vi "Run.vi"(7 "Team Index":i32, 8 "Column":i32, 9 "Row":i32, 10 "View":i32[](array[numeric]) caption="View (Team Index, -1: empty)", 11 "Impenetrable In":refnum<class "Impenetrable.lvclass">) -> (0 "Replicated":refnum<class "Square.lvclass">, 1 "Direction":T1, 2 "Action":T2, 3 "Square Out":refnum<class "Square.lvclass">)   [LabVIEW 2015, in "Impenetrable.lvclass"]
uses:
  Impenetrable.lvclass
  Square/Square.lvclass
  Type Defs/Action Enum.ctl
  Type Defs/Direction Enum.ctl
  Impenetrable.lvclass/Impenetrable.ctl
  Assassin/Assassin.lvclass
  Type.ctl
  SubVIs/Read-Only Globals.vi
  Common/Find Enemy.vi
  SubVIs/Globals (private).vi
  Globals.vi
  Common/Common.lvlib
  Type Defs/SB Type Defs.lvlib
panel:
  # "NW\nN\nNE\nE\nSE\nS\nSW\nW"
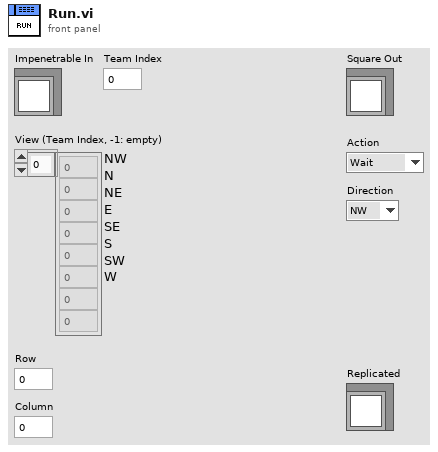
[diagram p1: front panel]
types:
  T1 = typedef "SB Type Defs.lvlib/Direction Enum.ctl" = enum16{"NW", "N", "NE", "E", "SE", "S", "SW", "W"}
  T2 = typedef "SB Type Defs.lvlib/Action Enum.ctl" = enum16{"Wait", "Move", "Attack", "Replicate"}
  T3 = typedef "Impenetrable.lvclass/Type.ctl" = enum16{"Assassin", "Starter", "Line Starter", "ELine", "WLine", "StartPatrol", "WPatrol", "EPatrol", "WWall", "EWall", "Rain"}
  T4 = typedef "Common.lvlib/Position.ctl" = cluster{"Column":i32, "Row":i32}
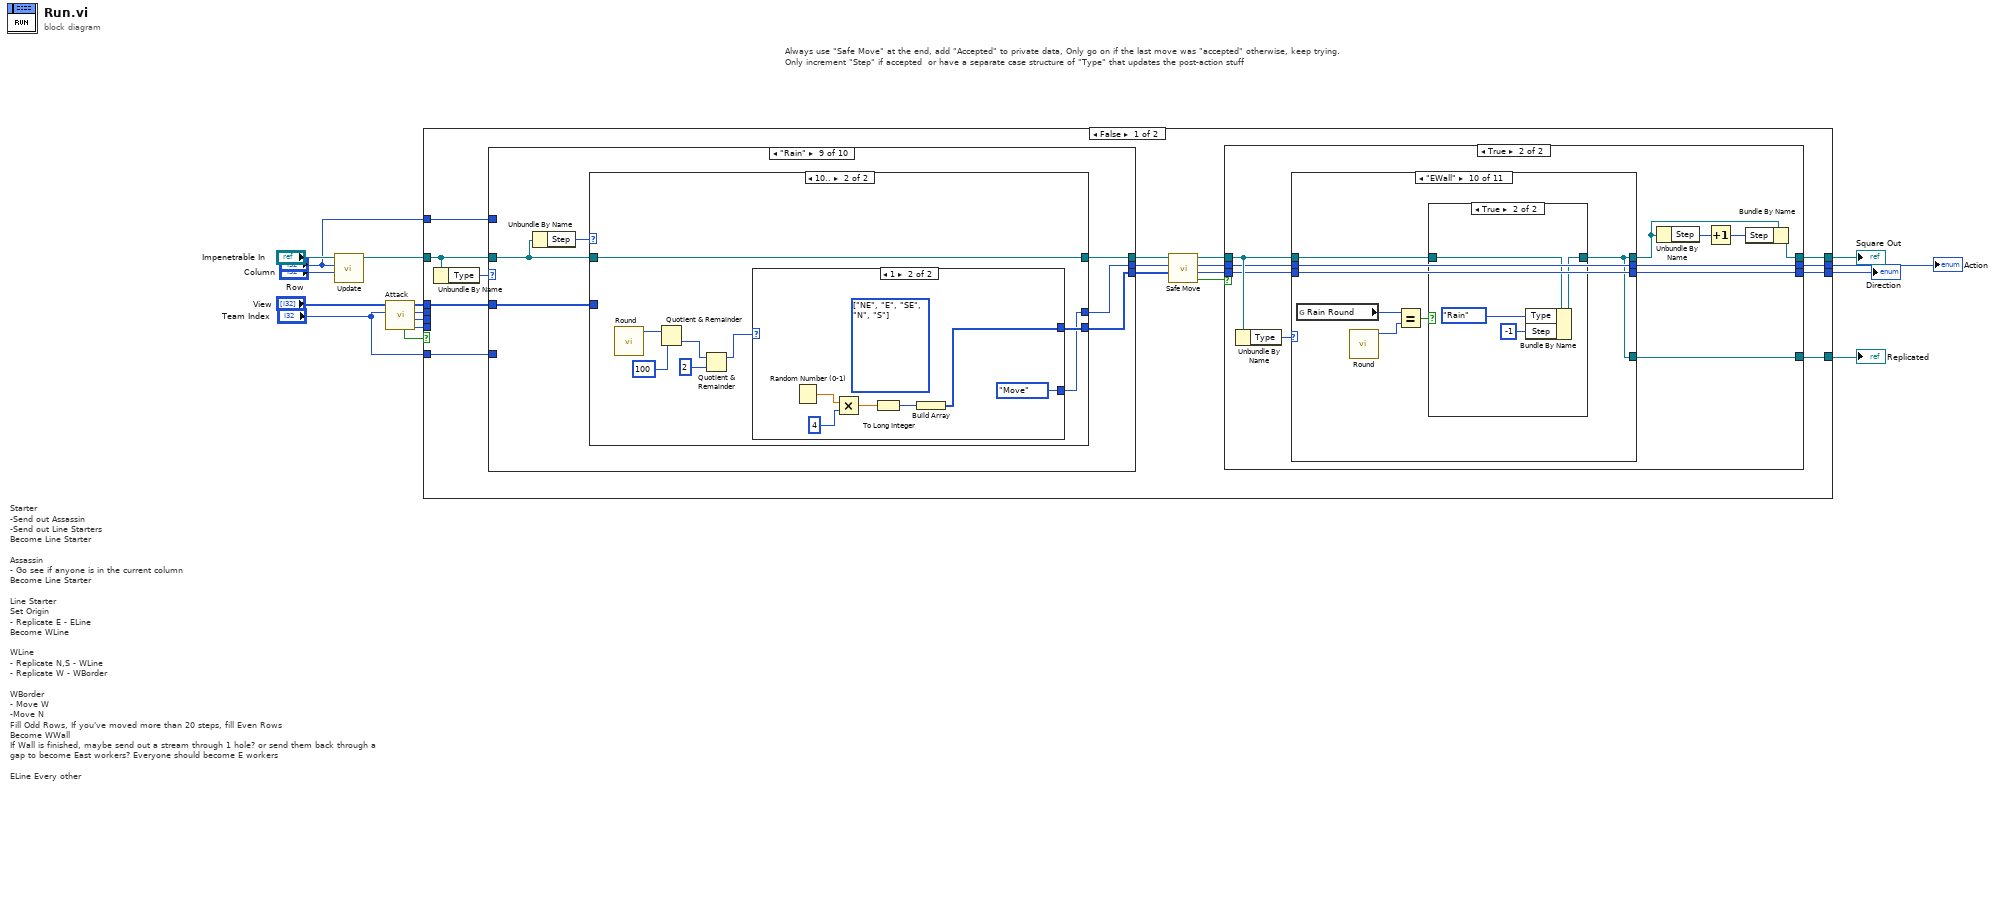
[diagram p0: block diagram]
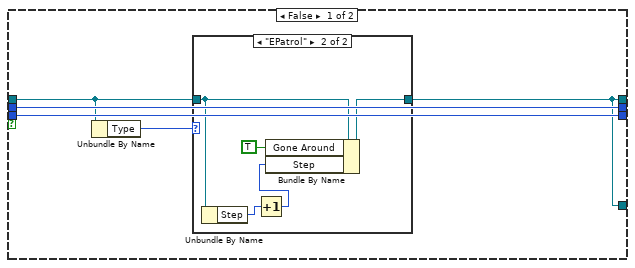
[diagram p2: hidden frame]
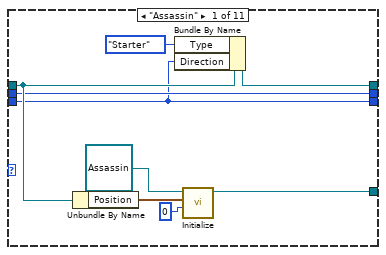
[diagram p4: hidden frame]
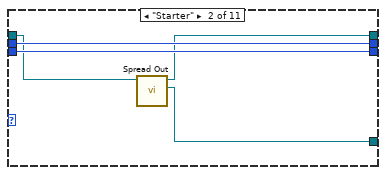
[diagram p5: hidden frame]
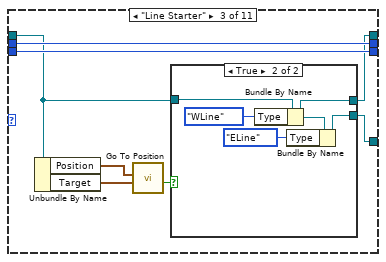
[diagram p6: hidden frame]
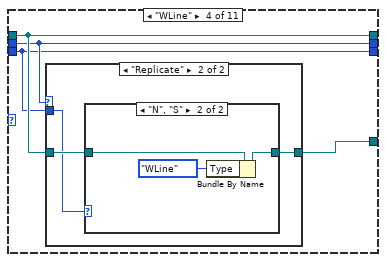
[diagram p8: hidden frame]
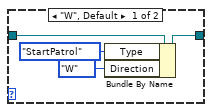
[diagram p10: hidden frame]
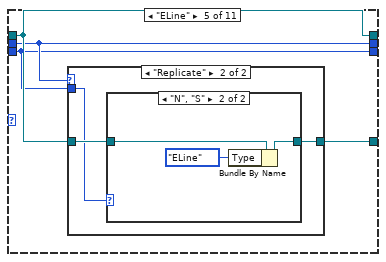
[diagram p11: hidden frame]
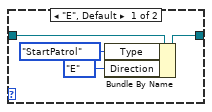
[diagram p13: hidden frame]
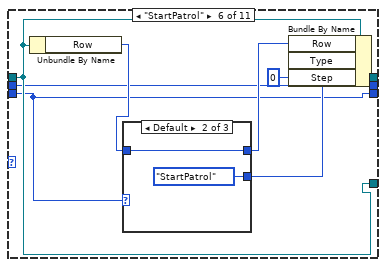
[diagram p14: hidden frame]
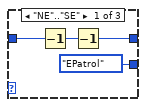
[diagram p15: hidden frame]
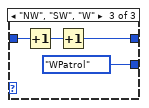
[diagram p16: hidden frame]
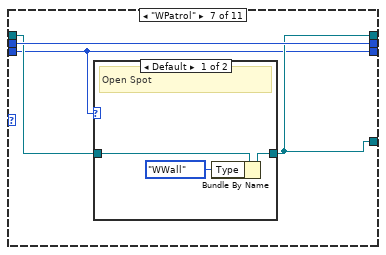
[diagram p17: hidden frame]
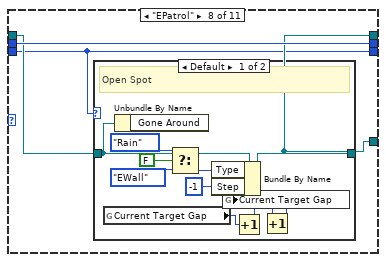
[diagram p19: hidden frame]
diagram:
  # "Always use \"Safe Move\" at the end, add \"Accepted\" to private data, Only go on if the last move was \"accepted\" otherwise, keep trying.\nOnly increment \"Step\" if accepted  or have a separate case structure of \"Type\" that updates the post-action stuff"
  # "Starter\n-Send out Assassin\n-Send out Line Starters\nBecome Line Starter\n\nAssassin\n- Go see if anyone is in the current column\nBecome Line Starter\n\nLine Starter\nSet Origin\n- Replicate E - ELine\nBecome WLine\n\nWLine\n- Replicate N,S - WLine\n- Replicate W - WBorder\n\nWBorder\n- Move W\n-Move N\nFill Odd Rows, If you've moved more than 20 steps, fill Even Rows\nBecome WWall\nIf Wall is finished, maybe send out a stream through 1 hole? or send them back through a gap to become East workers? Everyone should become E workers\n\nELine Every other"
  n1 = call "Update.vi"("Column"="Column", "Row"="Row", "Impenetrable In"="Impenetrable In") -> ("Impenetrable Out"=w12:refnum<class "Impenetrable.lvclass">)  [unwired: 8 in]
  n2 = call "Attack.vi"("Team Index"="Team Index", "View"="View") -> ("Enemy"=w5:i32, "Direction"=w6:i32, "Action"=w7:T2, "View"=w8:i32[], "Enemy Found?"=w10:bool)  [unwired: 4 in, 1 out]
  n3 = case shown="False" w10 {
    tunnel: [w16 w266] -> w13
    tunnel: [w27 w266] -> w4
    tunnel: w8 -> [w31 _]
    tunnel: "Team Index" -> [w30 _]
    tunnel: w12 -> [w29 w266]
    tunnel: w7 -> [_ w265]
    tunnel: w6 -> [_ w264]
    tunnel: w5 -> [_ _]
    tunnel: "Row" -> [w26 _]
    tunnel: [w20 w265] -> w2
    tunnel: [w19 w264] -> w1
    frame False {
      n4 = Unbundle By Name(w29) -> ("Type"=w28:T3)
      n5 = case shown="\"Rain\"" w28 {
        tunnel: w29 -> [w171 w178 w183 w200 w205 w206 w217 w221 w228 w262]
        tunnel: [w171 w178 w182 w200 w205 w206 w216 w221 w227 w262] -> w25
        tunnel: [Action_Enum."Replicate" ("Action") Action_Enum."Replicate" ("Action") w181 Action_Enum."Replicate" ("Desired Action") Action_Enum."Replicate" ("Desired Action") Action_Enum."Move" ("Action") Action_Enum."Move" ("Action") Action_Enum."Move" ("Action") w230 Action_Enum."Attack" ("Action")] -> w18
        tunnel: [w172 w179 w180 w201 w204 w207 w215 w220 w225 w260] -> w17
        tunnel: w31 -> [_ _ _ _ _ _ _ _ w226 _]
        tunnel: w30 -> [_ _ _ _ _ _ _ _ _ _]
        tunnel: w26 -> [_ _ _ _ _ _ _ _ _ _]
        frame "Assassin" {
          n6 = Unbundle By Name(w171) -> ("Direction"=w174:T1)
          n7 = call "Reverse Direction.vi"("Direction in"=w174) -> ("Reverse Direction"=w173:i32)  [unwired: 10 in]
          n8 = Build Array(w173) -> (w172:i32[])
        }
        frame "Starter" {
          n9 = Build Array(Direction_Enum."NE" ("Direction")) -> (w179:T1[])
        }
        frame "Line Starter" {
          n10 = Unbundle By Name(w183) -> ("Position"=w187:T4, "Target"=w186:T4)
          n11 = call "Go To Position.vi"("Target Position"=w186, "My Position"=w187) -> ("Arrived?"=w184:bool, "Direction"=w185:T1)  [unwired: 7 in, 1 out]
          n12 = case shown="False" w184 {
            tunnel: w183 -> [w195 w199]
            tunnel: [w195 w199] -> w182
            tunnel: [Action_Enum."Move" ("Action") Action_Enum."Replicate" ("Action")] -> w181
            tunnel: w185 -> [w192 _]
            tunnel: [w193 w196] -> w180
            frame False {
              n13 = call "CW Direction Shift.vi"("Direction"=w192) -> ("Numeric"=w191:i32)  [unwired: 10 in]
              n14 = call "CCW Direction Shift.vi"("Direction"=w192) -> ("Numeric"=w190:i32)  [unwired: 10 in]
              n15 = call "CCW Direction Shift.vi"("Direction"=w190) -> ("Numeric"=w188:i32)  [unwired: 10 in]
              n16 = call "CW Direction Shift.vi"("Direction"=w191) -> ("Numeric"=w189:i32)  [unwired: 10 in]
              n17 = Build Array(w192, w191, w190, w189, w188) -> (w193:i32[])
            }
            frame True {
              n18 = Build Array(Direction_Enum."E" ("Direction")) -> (w196:T1[])
            }
          }
        }
        frame "WLine" {
          w201 = T1[] [enum."S", enum."N", enum."W"] items=["NW", "N", "NE", "E", "SE", "S", "SW", "W"]
        }
        frame "ELine" {
          w204 = T1[] [enum."S", enum."N", enum."E"] items=["NW", "N", "NE", "E", "SE", "S", "SW", "W"]
        }
        frame "StartPatrol" {
          n19 = Unbundle By Name(w206) -> ("Direction"=w210:T1)
          n20 = call "CCW Direction Shift.vi"("Direction"=w210) -> ("Numeric"=w209:i32)  [unwired: 10 in]
          n21 = call "CW Direction Shift.vi"("Direction"=w210) -> ("Numeric"=w211:i32)  [unwired: 10 in]
          n22 = Build Array(w211, w210, w209) -> (w207:i32[])
        }
        frame "EPatrol" {
          # "W and S\nor\nE and N"
          n23 = call "Gone Around.vi"("Impenetrable in"=w217) -> ("Impenetrable out"=w216:refnum<class "Impenetrable.lvclass">)  [unwired: 10 in]
          n24 = Unbundle By Name(w216) -> ("Direction"=w213:T1)
          n25 = call "CW Direction Shift.vi"("Direction"=w213) -> ("Numeric"=w214:i32)  [unwired: 10 in]
          n26 = call "CW Direction Shift.vi"("Direction"=w214) -> ("Numeric"=w212:i32)  [unwired: 10 in]
          n27 = Build Array(w213, w212) -> (w215:i32[])
        }
        frame "WPatrol" {
          n28 = Unbundle By Name(w221) -> ("Direction"=w223:T1)
          n29 = call "CW Direction Shift.vi"("Direction"=w223) -> ("Numeric"=w224:i32)  [unwired: 10 in]
          n30 = call "CW Direction Shift.vi"("Direction"=w224) -> ("Numeric"=w222:i32)  [unwired: 10 in]
          n31 = Build Array(w223, w222) -> (w220:i32[])
        }
        frame "Rain" {
          n32 = Unbundle By Name(w228) -> ("Step"=w229:i32)
          n33 = case shown="10.." w229 {
            tunnel: [Action_Enum."Move" ("Action") w235] -> w230
            tunnel: [w231 w236] -> w225
            tunnel: [w232 w242] -> w227
            tunnel: w228 -> [w232 w242]
            tunnel: w226 -> [_ _]
            frame ..9 {
              n34 = Build Array(Direction_Enum."E" ("Direction")) -> (w231:T1[])
            }
            frame 10.. {
              n35 = call "Round.vi"() -> ("Round"=w241:i32)  [unwired: 11 in]
              n36 = Quotient & Remainder(x=w241, y=100) -> (floor(x/y)=w237:i32)  [unwired: 1 out]
              n37 = Quotient & Remainder(x=w237, y=2) -> (x-y*floor(x/y)=w238:i32)  [unwired: 1 out]
              n38 = case shown="1" w238 {
                tunnel: [w250 w254] -> w236
                tunnel: [w243 Action_Enum."Move" ("t")] -> w235
                frame 0, Default {
                  n39 = Random Number (0-1)() -> (number: 0 to 1=w253:dbl)
                  n40 = Multiply(x=w253, y=4) -> (x*y=w251:dbl)
                  n41 = Random Number (0-1)() -> (number: 0 to 1=w245:dbl)
                  n42 = To Long Integer(number=w251) -> (32bit integer=w249:i32)
                  n43 = Build Array(w249) -> (w250:i32[])
                  n44 = Greater?(x=w245, y=0.4 ("x")) -> (0:w247:bool)
                  n45 = Select(t=Action_Enum."Move", s=w247, f=Action_Enum."Replicate" ("t")) -> (s? t:f=w243:T2)
                }
                frame 1 {
                  (unwired) T1[] [enum."NE", enum."E", enum."SE", enum."N", enum."S"] items=["NW", "N", "NE", "E", "SE", "S", "SW", "W"]
                  n46 = Random Number (0-1)() -> (number: 0 to 1=w258:dbl)
                  n47 = Multiply(x=w258, y=4) -> (x*y=w256:dbl)
                  n48 = To Long Integer(number=w256) -> (32bit integer=w255:i32)
                  n49 = Build Array(w255) -> (w254:i32[])
                }
              }
            }
          }
        }
        frame "WWall", "EWall" {
          n50 = Unbundle By Name(w262) -> ("Direction"=w261:T1)
          n51 = Build Array(w261) -> (w260:T1[])
        }
      }
      n52 = call "Safe Move.vi"("Directions in"=w17, "Action in"=w18, "Impenetrable in"=w25) -> ("Accepted?"=w23:bool, "Direction"=w22:T1, "Action out"=w21:T2, "Impenetrable out"=w24:refnum<class "Impenetrable.lvclass">)  [unwired: 5 in]
      n53 = case shown="True" w23 {
        tunnel: [w34 w53] -> w27
        tunnel: w24 -> [w33 w49]
        tunnel: w22 -> [w35 w47]
        tunnel: w21 -> [w36 w46]
        tunnel: [w36 w45] -> w20
        tunnel: [w35 w44] -> w19
        tunnel: [w34 w50] -> w16
        frame False {
          n54 = Unbundle By Name(w33) -> ("Type"=w32:T3)
          n55 = case shown="\"EPatrol\"" w32 {
            tunnel: w33 -> [w37 w40]
            tunnel: [w37 w42] -> w34
            frame Default {
            }
            frame "EPatrol" {
              n56 = Unbundle By Name(w40) -> ("Step"=w39:i32)
              n57 = Increment(x=w39) -> (x+1=w38:i32)
              n58 = Bundle By Name(cluster=w40, "Gone Around"=TRUE, "Step"=w38) -> (w42:refnum<class "Impenetrable.lvclass">)
            }
          }
        }
        frame True {
          n59 = Unbundle By Name(w49) -> ("Type"=w48:T3)
          n60 = case shown="\"EWall\"" w48 {
            tunnel: w49 -> [w58 w65 w70 w84 w99 w115 w132 w140 w153 w160 w168]
            tunnel: [w59 w63 w68 w85 w100 w115 w131 w139 w153 w156 w168] -> w50
            tunnel: [w57 w64 w69 w84 w99 w119 w131 w139 w153 w156 w168] -> w43
            tunnel: w47 -> [w55 w66 w74 w82 w97 w113 w130 w138 w154 w161 w169]
            tunnel: w46 -> [w56 w67 w75 w83 w98 w114 w133 w141 w155 w162 w170]
            tunnel: [w56 w67 w75 w83 w98 w114 w133 w141 w155 w162 w170] -> w45
            tunnel: [w55 w66 w74 w82 w97 w113 w130 w138 w154 w161 w169] -> w44
            frame "Assassin" {
              n61 = Unbundle By Name(w58) -> ("Position"=w61:T4)
              n62 = Bundle By Name(cluster=w58, "Type"=Type."Starter", "Direction"=w55) -> (w57:refnum<class "Impenetrable.lvclass">)
              n63 = call "Initialize.vi"("Current Target"=0, "Position"=w61, "Assassin in"=refnum<class "Assassin.lvclass"> refnum ("Assassin.lvclass")) -> ("Assassin out"=w59:refnum<class "Assassin.lvclass">)  [unwired: 8 in]
            }
            frame "Starter" {
              n64 = call "Spread Out.vi"("Impenetrable in"=w65) -> ("64 out"=w63:refnum<class "Impenetrable.lvclass">, "Impenetrable out"=w64:refnum<class "Impenetrable.lvclass">)  [unwired: 9 in]
            }
            frame "Line Starter" {
              n65 = Unbundle By Name(w70) -> ("Position"=w73:T4, "Target"=w72:T4)
              n66 = call "Go To Position.vi"("Target Position"=w72, "My Position"=w73) -> ("Arrived?"=w71:bool)  [unwired: 7 in, 2 out]
              n67 = case shown="True" w71 {
                tunnel: w70 -> [w76 w81]
                tunnel: [w76 w79] -> w69
                tunnel: [w76 w78] -> w68
                frame False {
                }
                frame True {
                  n68 = Bundle By Name(cluster=w81, "Type"=Type."WLine") -> (w79:refnum<class "Impenetrable.lvclass">)
                  n69 = Bundle By Name(cluster=w79, "Type"=Type."ELine") -> (w78:refnum<class "Impenetrable.lvclass">)
                }
              }
            }
            frame "WLine" {
              n70 = case shown="\"Replicate\"" w83 {
                tunnel: [w86 w89] -> w85
                tunnel: w84 -> [w86 w88]
                tunnel: w82 -> [_ w87]
                frame "Wait", Default {
                }
                frame "Replicate" {
                  n71 = case shown="\"N\", \"S\"" w87 {
                    tunnel: w88 -> [w93 w96]
                    tunnel: [w92 w95] -> w89
                    frame "W", Default {
                      n72 = Bundle By Name(cluster=w93, "Type"=Type."StartPatrol", "Direction"=Direction_Enum."W") -> (w92:refnum<class "Impenetrable.lvclass">)
                    }
                    frame "N", "S" {
                      n73 = Bundle By Name(cluster=w96, "Type"=Type."WLine") -> (w95:refnum<class "Impenetrable.lvclass">)
                    }
                  }
                }
              }
            }
            frame "ELine" {
              n74 = case shown="\"Replicate\"" w98 {
                tunnel: [w101 w104] -> w100
                tunnel: w99 -> [w101 w103]
                tunnel: w97 -> [_ w102]
                frame "Wait", Default {
                }
                frame "Replicate" {
                  n75 = case shown="\"N\", \"S\"" w102 {
                    tunnel: w103 -> [w108 w111]
                    tunnel: [w107 w110] -> w104
                    frame "E", Default {
                      n76 = Bundle By Name(cluster=w108, "Type"=Type."StartPatrol", "Direction"=Direction_Enum."E") -> (w107:refnum<class "Impenetrable.lvclass">)
                    }
                    frame "N", "S" {
                      n77 = Bundle By Name(cluster=w111, "Type"=Type."ELine") -> (w110:refnum<class "Impenetrable.lvclass">)
                    }
                  }
                }
              }
            }
            frame "StartPatrol" {
              n78 = Unbundle By Name(w115) -> ("Row"=w118:i32)
              n79 = case shown="Default" w113 {
                tunnel: [Type."EPatrol" ("Type") Type."StartPatrol" ("f") Type."WPatrol" ("f")] -> w116
                tunnel: w118 -> [w121 w125 w128]
                tunnel: [w120 w125 w127] -> w117
                frame "NE".."SE" {
                  n80 = Decrement(x=w121) -> (x-1=w122:i32)
                  n81 = Decrement(x=w122) -> (x-1=w120:i32)
                }
                frame Default {
                }
                frame "NW", "SW", "W" {
                  n82 = Increment(x=w128) -> (x+1=w126:i32)
                  n83 = Increment(x=w126) -> (x+1=w127:i32)
                }
              }
              n84 = Bundle By Name(cluster=w115, "Row"=w117, "Type"=w116, "Step"=0) -> (w119:refnum<class "Impenetrable.lvclass">)
            }
            frame "WPatrol" {
              n85 = case shown="Default" w130 {
                tunnel: w132 -> [w135 w137]
                tunnel: [w136 w137] -> w131
                frame Default {
                  # "Open Spot"
                  n86 = Bundle By Name(cluster=w135, "Type"=Type."WWall") -> (w136:refnum<class "Impenetrable.lvclass">)
                }
                frame "N", "S" {
                  # "Patrol"
                }
              }
            }
            frame "EPatrol" {
              n87 = case shown="Default" w138 {
                tunnel: w140 -> [w147 w152]
                tunnel: [w151 w152] -> w139
                frame Default {
                  # "Open Spot"
                  n88 = global read "Globals.vi" "Current Target Gap"() -> (w144:i32)
                  n89 = Unbundle By Name(w147) -> ()  [unwired: 1 out]
                  n90 = Select(t=Type."Rain", s=FALSE, f=Type."EWall" ("Type")) -> (s? t:f=w149:T3)
                  n91 = Bundle By Name(cluster=w147, "Type"=w149, "Step"=-1) -> (w151:refnum<class "Impenetrable.lvclass">)
                  n92 = Increment(x=w144) -> (x+1=w145:i32)
                  n93 = Increment(x=w145) -> (x+1=w143:i32)
                  n94 = global write "Globals.vi" "Current Target Gap"(w143) -> ()
                }
                frame "N", "S" {
                  # "Patrol"
                }
              }
            }
            frame "WWall" {
            }
            frame "EWall" {
              n95 = global read "Globals.vi" "Rain Round"() -> (w159:i32)
              n96 = call "Round.vi"() -> ("Round"=w158:i32)  [unwired: 11 in]
              n97 = Equal?(x=w159, y=w158) -> (x = y?=w157:bool)
              n98 = case shown="True" w157 {
                tunnel: w160 -> [w163 w167]
                tunnel: [w163 w166] -> w156
                frame False {
                }
                frame True {
                  n99 = Bundle By Name(cluster=w167, "Type"=Type."Rain", "Step"=-1) -> (w166:refnum<class "Impenetrable.lvclass">)
                }
              }
            }
            frame "Rain" {
            }
          }
          n100 = Unbundle By Name(w43) -> ("Step"=w52:i32)
          n101 = Increment(x=w52) -> (x+1=w51:i32)
          n102 = Bundle By Name(cluster=w43, "Step"=w51) -> (w53:refnum<class "Impenetrable.lvclass">)
        }
      }
    }
    frame True {
    }
  }
  "Square Out" <- w4
  "Action" <- w2
  "Direction" <- w1
  "Replicated" <- w13
